vi "Send Msg.vi"(7 "Module":T1, 8 "error in (no error)":errorcluster, 9 "Message Data":variant, 10 "Message":string, 11 "Module Routes":refnum<user-event>[](array[refnum])) -> (0 "error out":errorcluster)   [LabVIEW 2018]
doc: "Send a message to one module"
uses:
  Modules.ctl
  Message Queue/Message Cluster.ctl
  Message Queue/Message Queue.lvlib
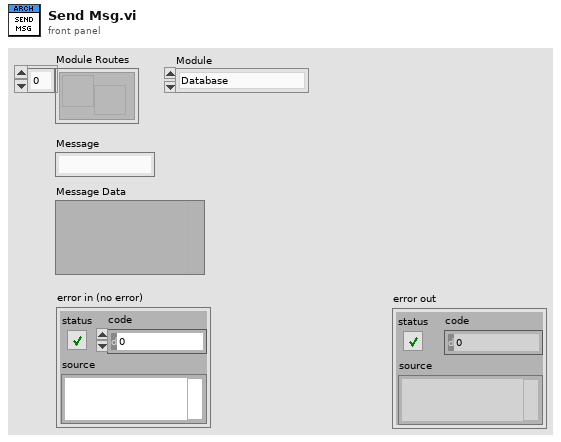
[diagram p1: front panel]
types:
  T1 = typedef "Modules.ctl" = enum16{"Database", "Car Wash Controller", "Console"}
  T2 = typedef "Message Queue.lvlib/Message Cluster.ctl" = cluster{"Message":string, "Message Data":variant}
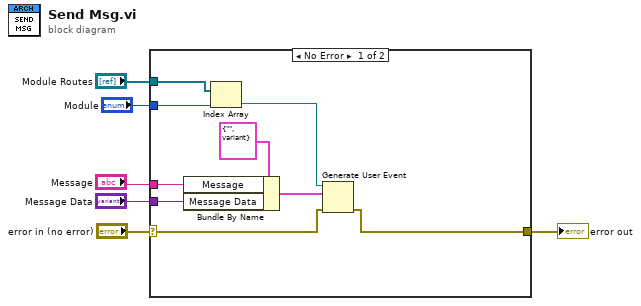
[diagram p0: block diagram]
diagram:
  n1 = case shown="No Error" "error in (no error)" {
    selector: "error in (no error)" -> [w11 w16]
    tunnel: "Module Routes" -> [w15 _]
    tunnel: "Module" -> [w14 _]
    tunnel: [w12 w16] -> w4
    tunnel: "Message" -> [w8 _]
    tunnel: "Message Data" -> [w7 _]
    frame No Error {
      n2 = Bundle By Name(cluster=T2 {"Message"="", "Message Data"=variant} ("event data"), "Message"=w8, "Message Data"=w7) -> (w9:T2)
      n3 = Index Array(array=w15, index=w14) -> (element=w13:refnum<user-event>)
      n4 = Generate User Event(user event=w13, event data cluster=w9, error in=w11) -> (error out=w12:errorcluster)  [unwired: 1 in, 1 out]
    }
    frame Error {
    }
  }
  "error out" <- w4
